vi "Create.vi"(10 "Module ID":string) -> (3 "GUI Identity out":refnum<class "GUI Identity.lvclass">)   [LabVIEW 2020, in "VolatusGUI.lvlib" / "GUI Identity.lvclass"]
uses:
  GUI Identity.lvclass
  GUI Identity.lvclass/GUI Identity.ctl
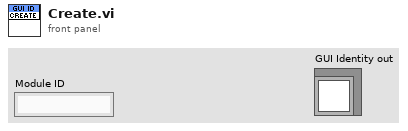
[diagram p1: front panel]
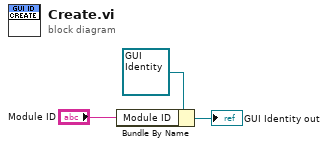
[diagram p0: block diagram]
diagram:
  n1 = Bundle By Name(cluster=refnum<class "GUI Identity.lvclass"> refnum ("GUI Identity in"), "Module ID"="Module ID") -> (→"GUI Identity out":refnum<class "GUI Identity.lvclass">)
